vi "Initialize File Writing.vi"(8 "error in":errorcluster, 11 "cPAS Facade in":refnum<class "cPAS Facade.lvclass">) -> (0 "error out":errorcluster, 3 "cPAS Facade out":refnum<class "cPAS Facade.lvclass">)   [LabVIEW 2015, in "cPAS Facade.lvclass"]
uses:
  cPAS Facade.lvclass
  Data.ctl
  Observer/File/cPAS File Obs.lvclass
  Observer/File/cCRDS/cCRDS File Obs.lvclass
  Devices/CLAP/Observers/File Writer/CLAP File Obs.lvclass
  Reusable/Observer/Observer.lvclass/Observer.ctl
  Reusable/File IO/Class/File Observer.lvclass/File Observer.ctl
  Reusable/GUI/Facade/GUI Facade.lvclass/GUI Facade.ctl
  Reusable/Observer/Write Data Queue.vi
  Reusable/File IO/Class/Accessors/Write Max Size.vi
  Reusable/File IO/Class/Accessors/Write Top Data Path.vi
  Reusable/File IO/Class/Write Write.vi
  Reusable/File IO/Class/Accessors/Write File Prefix.vi
  Reusable/File IO/Class/Accessors/Write File Ext.vi
  Reusable/GUI/Facade/GUI Facade.lvclass
  Reusable/File IO/Class/File Observer.lvclass
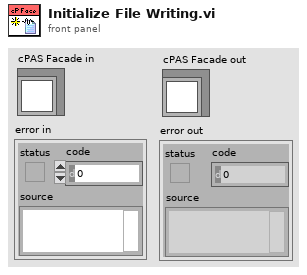
[diagram p1: front panel]
types:
  T1 = typedef "cPAS Facade.lvclass/Data.ctl" = enum16{"PAS", "CRD", "CLAP"}
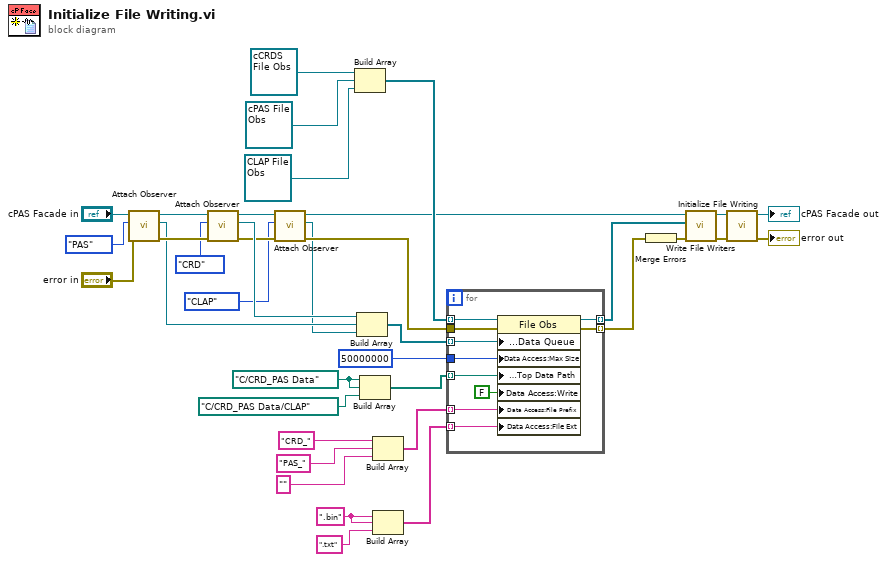
[diagram p0: block diagram]
diagram:
  w13 = ".bin" ("File Ext")
  w17 = path "C:/CRD_PAS Data" ("Top Data Path")
  n1 = call "Attach Observer.vi"("error in"="error in", "Subject"=Data."PAS" ("Data"), "GUI Facade in"="cPAS Facade in") -> ("error out"=w33:errorcluster, "Observer"=w29:refnum<queue>, "GUI Facade out"=w32:refnum<class "cPAS Facade.lvclass">)  [unwired: 6 in]
  n2 = call "Attach Observer.vi"("error in"=w33, "Subject"=Data."CRD" ("Data"), "GUI Facade in"=w32) -> ("error out"=w9:errorcluster, "Observer"=w30:refnum<queue>, "GUI Facade out"=w10:refnum<class "cPAS Facade.lvclass">)  [unwired: 6 in]
  n3 = call "Attach Observer.vi"("error in"=w9, "Subject"=Data."CLAP" ("Data"), "GUI Facade in"=w10) -> ("error out"=w8:errorcluster, "Observer"=w7:refnum<queue>, "GUI Facade out"=w5:refnum<class "cPAS Facade.lvclass">)  [unwired: 6 in]
  n4 = Build Array(refnum<class "cCRDS File Obs.lvclass"> refnum ("cCRDS File Obs"), refnum<class "cPAS File Obs.lvclass"> refnum ("cPAS File Obs"), refnum<class "CLAP File Obs.lvclass"> refnum ("CLAP File Obs")) -> (w24:refnum<class "File Observer.lvclass">[])
  n5 = Build Array(w30, w29, w7) -> (w28:refnum<queue>[])
  n6 = Build Array(w17, w17, path "C:/CRD_PAS Data/CLAP" ("Top Data Path")) -> (w14:path[])
  n7 = Build Array("CRD_" ("element"), "PAS_" ("File Prefix"), "" ("element")) -> (w25:string[])
  n8 = Build Array(w13, w13, ".txt" ("element")) -> (w11:string[])
  n9 = for {
    tunnel: w28 -> [w47] mode=indexing
    tunnel: w25 -> [w46] mode=indexing
    tunnel: w24 -> [w44] mode=indexing
    tunnel: w8 -> [w43]
    tunnel: w14 -> [w42] mode=indexing
    tunnel: i64 50000000 ("Max Size") -> [w41]
    tunnel: [w40] -> w21 mode=indexing
    tunnel: [w39] -> w3 mode=indexing
    tunnel: w11 -> [w38] mode=indexing
    n10 = property class="File Obs"(reference=w44, error in=w43, "Data Access:Data Queue"=w47, "Data Access:Max Size"=w41, "Data Access:Top Data Path"=w42, "Data Access:Write"=FALSE ("Write"), "Data Access:File Prefix"=w46, "Data Access:File Ext"=w38) -> (reference out=w39:refnum<class "File Observer.lvclass">, error out=w40:errorcluster)
  }
  n11 = Merge Errors(w21) -> (w2:errorcluster)
  n12 = call "Write File Writers.vi"("error in"=w2, "File Writers"=w3, "GUI Facade in"=w5) -> ("error out"=w1:errorcluster, "GUI Facade out"=w4:refnum<class "cPAS Facade.lvclass">)  [unwired: 7 in]
  n13 = call-parent "Initialize File Writing.vi"("error in"=w1, "GUI Facade in"=w4) -> ("error out"=→"error out":errorcluster, "GUI Facade out"=→"cPAS Facade out":refnum<class "cPAS Facade.lvclass">)  [unwired: 8 in]
